vi "Base Card Passthrough(SLSC Switch).vi"(4 "Iterations":u32=50 min=1 max=64, 6 "Channels (1-64)":u16=64 min=1 max=64, 9 "Disconnection":T2(ring)=enum."Disconnect Single", 10 "Connection":enum16{"Connect Single", "Connect Array"}(ring)=enum."Connect Array", 11 "device":refnum<k21>="SET-2010-Mod2") -> (0 "error out":errorcluster, 1 "Disconnect Timing":T1, 2 "Connect Timing":T1)   [LabVIEW 2020, in "slsc-switch-benchmarks.lvlib"]
uses:
  slsc-switch-benchmarks.lvlib
  Timing Statistics.ctl
  <vilib>/SLSC_Switch/Initialize with Topology (Override Switches).vi
  <vilib>/SLSC_Switch/Connect Channels (Single).vi
  <vilib>/SLSC_Switch/Connect Channels (Multiple).vi
  <vilib>/SLSC_Switch/Disconnect Channels (Single).vi
  <vilib>/SLSC_Switch/Disconnect Channels (Multiple).vi
  <vilib>/SLSC_Switch/SLSC Switch.lvlib
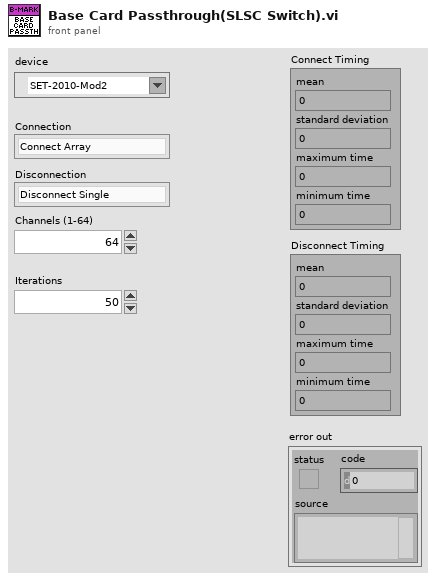
[diagram p1: front panel]
types:
  T1 = typedef "slsc-switch-benchmarks.lvlib/Timing Statistics.ctl" = cluster{"mean":dbl, "standard deviation":dbl, "maximum time":dbl, "minimum time":dbl}
  T2 = enum16{"No-Op", "Disconnect Single", "Disconnect Array", "Disconnect All"}
  T3 = cluster{"Connect Time":dbl, "Disconnect Time":dbl}
  T4 = cluster{"Source Channel":string, "Destination Channel":string}[]
  T5 = typedef "nislscslSession.ctl" = refnum<k20>
  T6 = cluster{"Connect Time":dbl, "Disconnect Time":dbl}[]
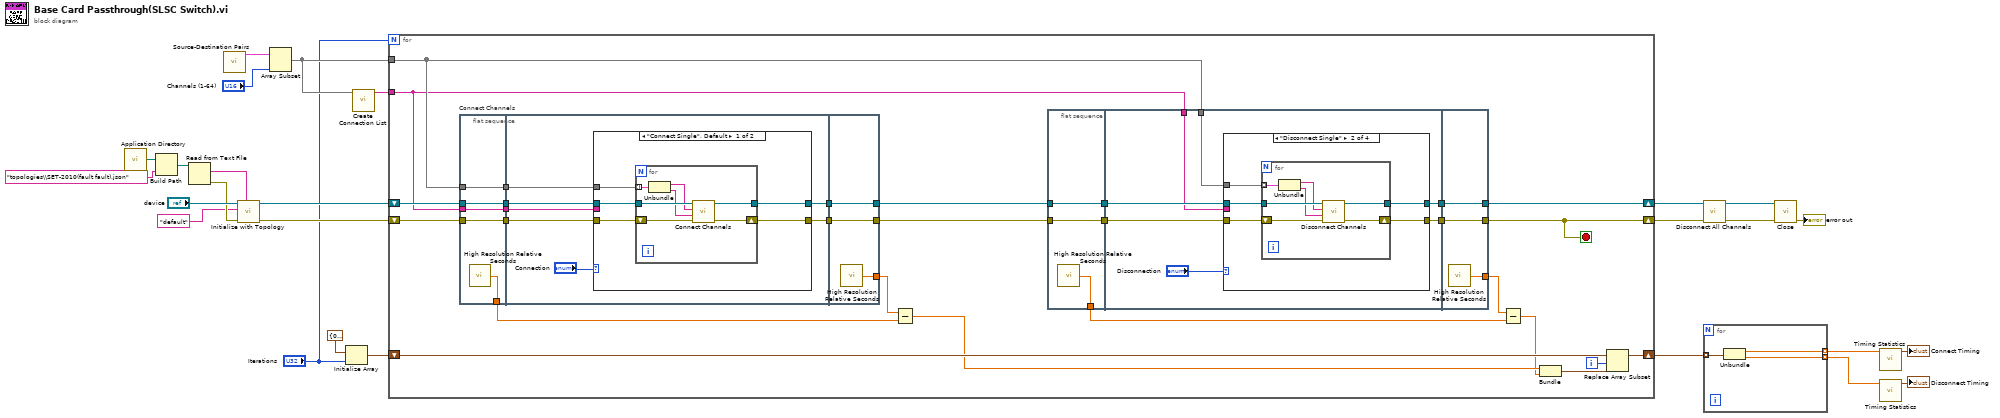
[diagram p0: block diagram]
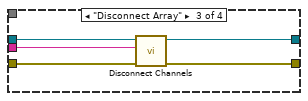
[diagram p3: hidden frame]
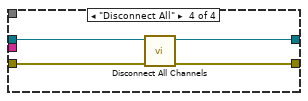
[diagram p4: hidden frame]
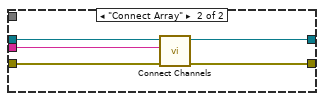
[diagram p5: hidden frame]
diagram:
  n1 = call <vilib>:"Application Directory.vi"() -> ("Application Directory"=w25:path)
  n2 = Build Path(base path=w25, name or relative path="topologies\\SET-2010(fault fault).json") -> (appended path=w23:path)
  n3 = Read from Text File(file (use dialog)=w23) -> (text=w21:string, error out=w22:errorcluster)  [unwired: 3 in, 2 out]
  n4 = call "Source-Destination Pairs.vi"() -> ("Source-Dest Pairs"=w19:T4)  [unwired: 11 in]
  n5 = call-poly <vilib>:"Initialize with Topology.vi"("switches json"=w21, "error in (no error)"=w22, "topology"="default", "device"="device") -> ("error out"=w16:errorcluster, "session out"=w17:T5)  [unwired: 6 in]
  n6 = Array Subset(array=w19, length="Channels (1-64)") -> (w14:T4)  [unwired: 1 in]
  n7 = Initialize Array(T3 {"Connect Time"=0.0, "Disconnect Time"=0.0}, "Iterations") -> (w10:T6)
  n8 = call "Create Connection List.vi"("Connection Pairs"=w14) -> ("Connection List"=w13:string)  [unwired: 10 in]
  n9 = for {
    N: "Iterations" -> [_]
    tunnel: w14 -> [w49]
    tunnel: w13 -> [w48]
    shift-right: [w50] -> w9
    shift-left: w17 -> [w54]
    shift-right: [w33] -> w8
    shift-left: w16 -> [w53]
    shift-right: [w30] -> w5
    shift-left: w10 -> [w31]
    i -> [w32]
    stop <- w33 stop-if-true
    n10 = flat-sequence "Connect Channels" {
      tunnel: w48 -> [w92]
      tunnel: w49 -> [w93]
      tunnel: w53 -> [w94]
      tunnel: w54 -> [w95]
      tunnel: [w95] -> w45
      tunnel: [w94] -> w44
      tunnel: [w93] -> w43
      tunnel: [w92] -> w42
      tunnel: [w91] -> w40
      tunnel: [w99] -> w47
      tunnel: [w98] -> w46
      tunnel: w45 -> [w102]
      tunnel: w44 -> [w101]
      tunnel: w43 -> [w97]
      tunnel: w42 -> [w96]
      tunnel: [w121] -> w51
      tunnel: [w122] -> w52
      tunnel: w47 -> [w122]
      tunnel: w46 -> [w121]
      tunnel: [w120] -> w41
      frame #0 {
        n11 = call <vilib>:"High Resolution Relative Seconds.vi"() -> ("relative seconds"=w91:dbl)
      }
      frame #1 {
        n12 = case shown="\"Connect Single\", Default" "Connection" {
          tunnel: w102 -> [w107 w119]
          tunnel: w101 -> [w106 w118]
          tunnel: w97 -> [w105 _]
          tunnel: [w104 w116] -> w98
          tunnel: [w103 w115] -> w99
          tunnel: w96 -> [_ w117]
          frame "Connect Single", Default {
            n13 = for {
              tunnel: w107 -> [w114]
              tunnel: w105 -> [w112] mode=indexing
              tunnel: [w109] -> w103
              shift-right: [w108] -> w104
              shift-left: w106 -> [w113]
              n14 = Unbundle(w112) -> ("Source Channel"=w110:string, "Destination Channel"=w111:string)
              n15 = call-poly <vilib>:"Connect Channels.vi"("error in (no error)"=w113, "channel 2"=w111, "channel 1"=w110, "session in"=w114) -> ("error out"=w108:errorcluster, "session out"=w109:T5)  [unwired: 6 in]
            }
          }
          frame "Connect Array" {
            n16 = call-poly <vilib>:"Connect Channels.vi"("error in (no error)"=w118, "connection list"=w117, "session in"=w119) -> ("error out"=w116:errorcluster, "session out"=w115:T5)  [unwired: 7 in]
          }
        }
      }
      frame #2 {
        n17 = call <vilib>:"High Resolution Relative Seconds.vi"() -> ("relative seconds"=w120:dbl)
      }
    }
    n18 = Subtract(x=w41, y=w40) -> (x-y=w29:dbl)
    n19 = flat-sequence {
      tunnel: w51 -> [w56]
      tunnel: w52 -> [w57]
      tunnel: [w57] -> w39
      tunnel: [w56] -> w38
      tunnel: [w55] -> w34
      tunnel: w49 -> [w59]
      tunnel: w48 -> [w58]
      tunnel: w39 -> [w64]
      tunnel: w38 -> [w63]
      tunnel: [w62] -> w37
      tunnel: [w61] -> w36
      tunnel: [w89] -> w50
      tunnel: [w90] -> w33
      tunnel: w37 -> [w90]
      tunnel: w36 -> [w89]
      tunnel: [w88] -> w35
      frame #0 {
        n20 = call <vilib>:"High Resolution Relative Seconds.vi"() -> ("relative seconds"=w55:dbl)
      }
      frame #1 {
        n21 = case shown="\"Disconnect Single\"" "Disconnection" {
          tunnel: w64 -> [w66 w70 w81 w86]
          tunnel: w63 -> [w65 w71 w83 w87]
          tunnel: [w65 w69 w82 w84] -> w62
          tunnel: [w66 w68 w80 w85] -> w61
          tunnel: w59 -> [_ w67 _ _]
          tunnel: w58 -> [_ _ w79 _]
          frame "No-Op", Default {
          }
          frame "Disconnect Single" {
            n22 = for {
              shift-right: [w76] -> w69
              shift-left: w71 -> [w78]
              tunnel: w70 -> [w77]
              tunnel: [w75] -> w68
              tunnel: w67 -> [w74] mode=indexing
              n23 = Unbundle(w74) -> ("Source Channel"=w72:string, "Destination Channel"=w73:string)
              n24 = call-poly <vilib>:"Disconnect Channels.vi"("error in (no error)"=w78, "channel 2"=w73, "channel 1"=w72, "session in"=w77) -> ("error out"=w76:errorcluster, "session out"=w75:T5)  [unwired: 6 in]
            }
          }
          frame "Disconnect Array" {
            n25 = call-poly <vilib>:"Disconnect Channels.vi"("error in (no error)"=w83, "disconnection list"=w79, "session in"=w81) -> ("error out"=w82:errorcluster, "session out"=w80:T5)  [unwired: 7 in]
          }
          frame "Disconnect All" {
            n26 = call <vilib>:"Disconnect All Channels.vi"("error in (no error)"=w87, "session in"=w86) -> ("error out"=w84:errorcluster, "session out"=w85:T5)  [unwired: 8 in]
          }
        }
      }
      frame #2 {
        n27 = call <vilib>:"High Resolution Relative Seconds.vi"() -> ("relative seconds"=w88:dbl)
      }
    }
    n28 = Subtract(x=w35, y=w34) -> (x-y=w28:dbl)
    n29 = Bundle(w29, w28) -> (w27:cluster{dbl, dbl})  [unwired: 1 in]
    n30 = Replace Array Subset(array=w31, new element=w27, index=w32) -> (w30:T6)
  }
  n31 = call <vilib>:"Disconnect All Channels.vi"("error in (no error)"=w8, "session in"=w9) -> ("error out"=w7:errorcluster, "session out"=w6:T5)  [unwired: 8 in]
  n32 = for {
    tunnel: w5 -> [w125] mode=indexing
    tunnel: [w124] -> w4 mode=indexing
    tunnel: [w123] -> w3 mode=indexing
    n33 = Unbundle(w125) -> ("Connect Time"=w124:dbl, "Disconnect Time"=w123:dbl)
  }
  n34 = call <vilib>:"Close.vi"("error in (no error)"=w7, "session in"=w6) -> ("error out"=→"error out":errorcluster)  [unwired: 9 in]
  n35 = call "Timing Statistics.vi"("Execution Speeds"=w4) -> ("Timing Statistics"=→"Connect Timing":T1)  [unwired: 10 in]
  n36 = call "Timing Statistics.vi"("Execution Speeds"=w3) -> ("Timing Statistics"=→"Disconnect Timing":T1)  [unwired: 10 in]
